vi "Set Exclude Tags.vi"(8 "error in (no error)":errorcluster, 11 "BuildSpec in":refnum<vi>) -> (0 "error out":errorcluster, 3 "BuildSpec out":refnum<vi>)   [LabVIEW 2019, in "Project Sync Tools.lvclass"]
uses:
  Project Sync Tools.lvclass
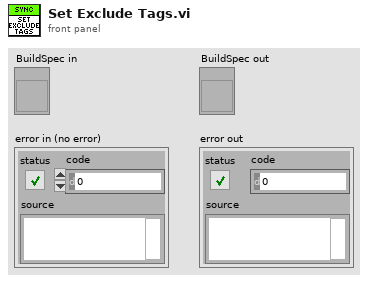
[diagram p1: front panel]
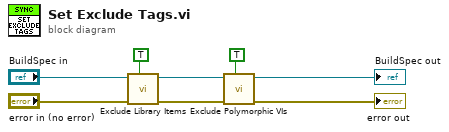
[diagram p0: block diagram]
diagram:
  n1 = call "Exclude Library Items.vi"("Exclude?"=TRUE ("Is Persistent (T)"), "error in (no error)"="error in (no error)", "BuildSpec in"="BuildSpec in") -> ("error out"=w3:errorcluster, "BuildSpec out"=w4:refnum<vi>)  [unwired: 7 in]
  n2 = call "Exclude Polymorphic VIs.vi"("Exclude ?"=TRUE, "error in (no error)"=w3, "BuildSpec in"=w4) -> ("error out"=→"error out":errorcluster, "BuildSpec out"=→"BuildSpec out":refnum<vi>)  [unwired: 7 in]
